vi "GoToBallSkillVSS.vi"(8 "error in (no error)":errorcluster, 9 "Game":refnum<class "Game.lvclass">, 10 "Robot in":refnum<class "Robot.lvclass">, 11 "GoToBallSkillVSS in":refnum<class "GoToBallSkillVSS.lvclass">) -> (0 "error out":errorcluster, 1 "Robot out":refnum<class "Robot.lvclass">, 3 "GoToBallSkillVSS out":refnum<class "GoToBallSkillVSS.lvclass">)   [LabVIEW 2020, in "GoToBallSkillVSS.lvclass"]
uses:
  GoToBallSkillVSS.lvclass
  Robot_class/Robot.lvclass
  C:/ROBOIME/SSL_AI/Object_class/Object.lvclass
  Game_class/Game.lvclass
  Object_class/Object.lvclass/Object.ctl
  Game_class/Game.lvclass/Game.ctl
  Robot_class/Robot.lvclass/Robot.ctl
  Game_class/Read BallRef.vi
  Object_class/Read x.vi
  Object_class/Read y.vi
  Robot_class/Write dest_orientation.vi
  Robot_class/Write dest_x.vi
  Robot_class/Write dest_y.vi
  Ball_class/Ball.lvclass
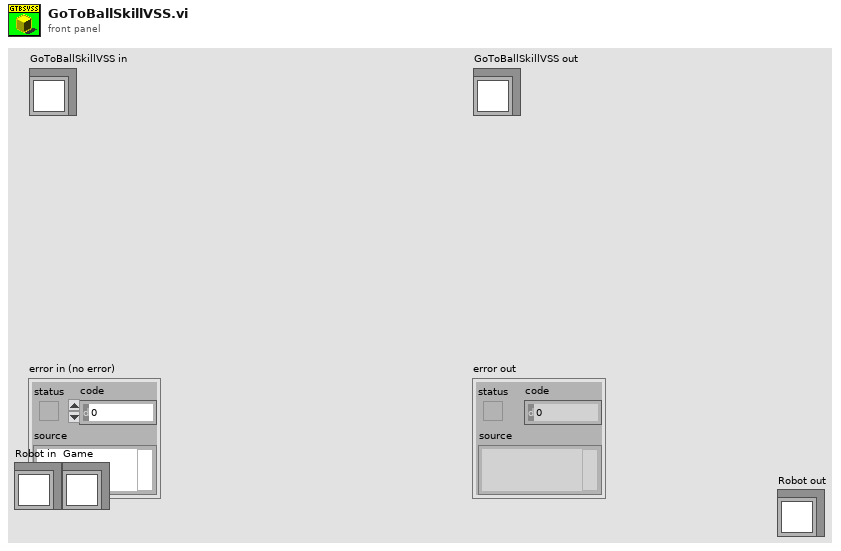
[diagram p1: front panel]
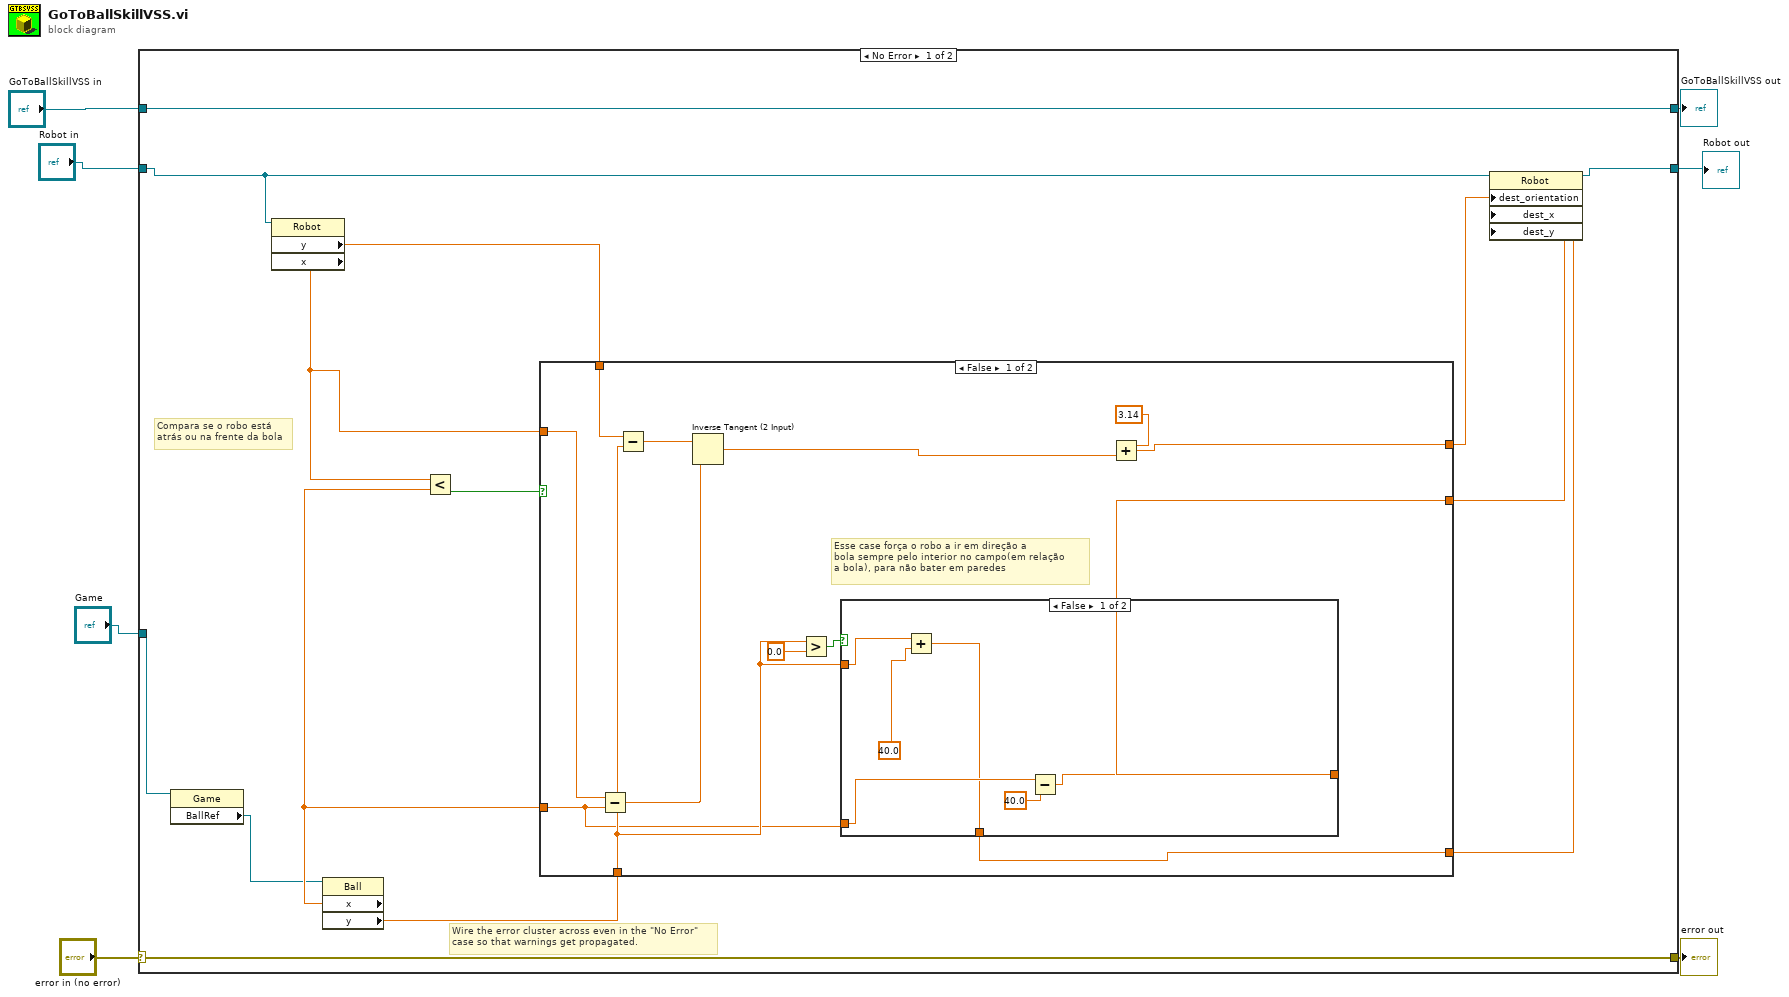
[diagram p0: block diagram]
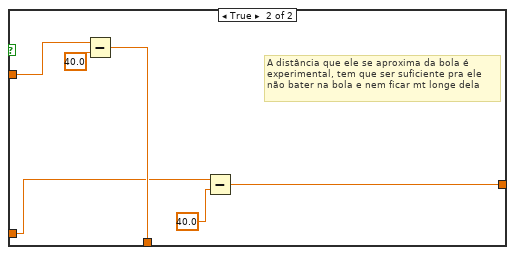
[diagram p2: hidden frame]
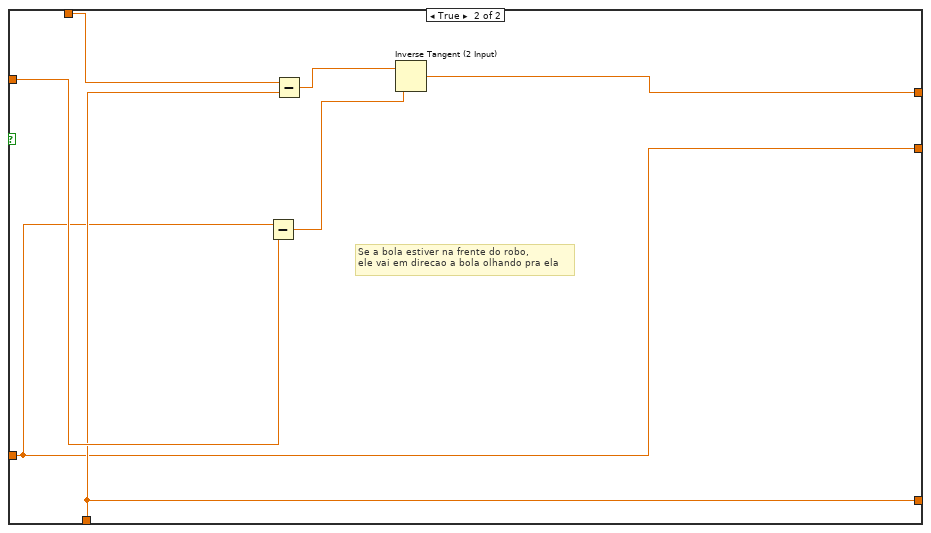
[diagram p3: hidden frame]
diagram:
  n1 = case shown="No Error" "error in (no error)" {
    selector: "error in (no error)" -> [w20 w56]
    tunnel: [w20 w56] -> w6
    tunnel: [w21 w55] -> w4
    tunnel: "GoToBallSkillVSS in" -> [w21 w55]
    tunnel: [w12 w54] -> w2
    tunnel: "Robot in" -> [w11 w54]
    tunnel: "Game" -> [w10 _]
    frame No Error {
      # "Compara se o robo está\natrás ou na frente da bola"
      # "Wire the error cluster across even in the \"No Error\"\ncase so that warnings get propagated."
      n2 = property class="Game"(reference=w10) -> ("BallRef"=w9:refnum<class "Ball.lvclass">)  [unwired: 1 in, 2 out]
      n3 = property class="Robot"(reference=w11) -> ("y"=w19:dbl, "x"=w16:dbl)  [unwired: 1 in, 2 out]
      n4 = property class="Ball"(reference=w9) -> ("x"=w17:dbl, "y"=w18:dbl)  [unwired: 1 in, 2 out]
      n5 = Less?(x=w16, y=w17) -> (x < y?=w8:bool)
      n6 = case shown="False" w8 {
        tunnel: [w30 w53] -> w15
        tunnel: w19 -> [w29 w50]
        tunnel: w18 -> [w25 w48]
        tunnel: w17 -> [w24 w47]
        tunnel: w16 -> [w28 w49]
        tunnel: [w23 w48] -> w14
        tunnel: [w22 w47] -> w13
        frame False {
          # "Esse case força o robo a ir em direção a \nbola sempre pelo interior no campo(em relação \na bola), para não bater em paredes"
          n7 = Subtract(x=w28, y=w24) -> (x-y=w33:dbl)
          n8 = Subtract(x=w29, y=w25) -> (x-y=w34:dbl)
          n9 = Inverse Tangent (2 Input)(1:w33, 2:w34) -> (0:w32:dbl)
          n10 = Greater?(x=w25, y=0.0) -> (0:w26:bool)
          n11 = case shown="False" w26 {
            tunnel: [w36 w46] -> w22
            tunnel: w25 -> [w39 w41]
            tunnel: w24 -> [w38 w42]
            tunnel: [w35 w43] -> w23
            frame False {
              n12 = Add(x=w39, y=40.0) -> (x+y=w35:dbl)
              n13 = Subtract(x=w38, y=40.0) -> (x-y=w36:dbl)
            }
            frame True {
              # "A distância que ele se aproxima da bola é\nexperimental, tem que ser suficiente pra ele \nnão bater na bola e nem ficar mt longe dela"
              n14 = Subtract(x=w41, y=40.0) -> (x-y=w43:dbl)
              n15 = Subtract(x=w42, y=40.0) -> (x-y=w46:dbl)
            }
          }
          n16 = Add(x=3.14, y=w32) -> (x+y=w30:dbl)
        }
        frame True {
          # "Se a bola estiver na frente do robo, \nele vai em direcao a bola olhando pra ela"
          n17 = Subtract(x=w47, y=w49) -> (x-y=w52:dbl)
          n18 = Subtract(x=w50, y=w48) -> (x-y=w51:dbl)
          n19 = Inverse Tangent (2 Input)(1:w52, 2:w51) -> (0:w53:dbl)
        }
      }
      n20 = property class="Robot"(reference=w11, "dest_orientation"=w15, "dest_x"=w13, "dest_y"=w14) -> (reference out=w12:refnum<class "Robot.lvclass">)  [unwired: 1 in, 1 out]
    }
    frame Error {
    }
  }
  "error out" <- w6
  "GoToBallSkillVSS out" <- w4
  "Robot out" <- w2
